vi "Collection demo.vi"() -> ()   [LabVIEW 2009]
uses:
  Minus/Minus.lvclass
  Collection.lvclass
  DAQ/DAQmx Analog.lvclass
  Lockin/Lockin SR830.lvclass
  Std Dev/Std Dev.lvclass
panel:
  out "error out":errorcluster
  in  "stop":bool
  out "Waveform Chart":waveform(dbl)[](graph)
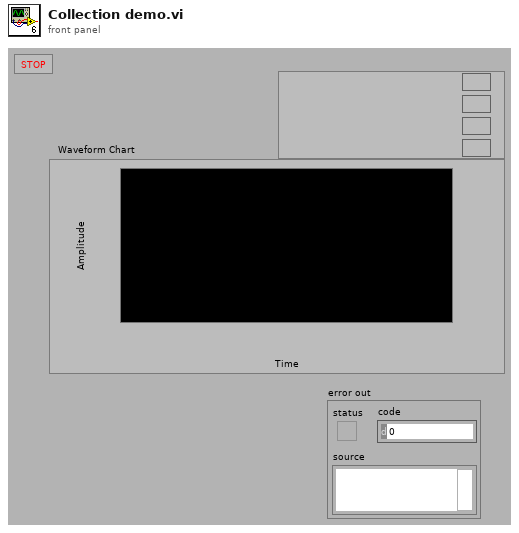
[diagram p1: front panel]
types:
  T1 = typedef "Readable.lvclass/TX Graph.ctl" = cluster{"Data Points":cluster{"t":timestamp, "x":dbl}[]}[]
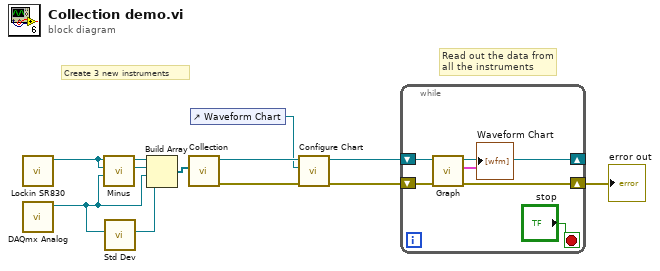
[diagram p0: block diagram]
diagram:
  # "Read out the data from\nall the instruments"
  # "Create 3 new instruments"
  n1 = call "Lockin SR830.vi"() -> ("Lockin SR830 out"=w3:refnum<class "Lockin SR830.lvclass">)  [unwired: 1 in, 10 out]
  n2 = call "DAQmx Analog.vi"() -> ("DAQmx Analog out"=w2:refnum<class "DAQmx Analog.lvclass">)  [unwired: 1 in, 10 out]
  n3 = call "Minus.vi"("Readable B"=w2, "Readable A"=w3) -> ("Minus.lvclass out"=w4:refnum<class "Minus.lvclass">)  [unwired: 1 in, 8 out]
  n4 = call "Std Dev.vi"("From"=w2) -> ("Std Dev.lvclass out"=w1:refnum<class "Std Dev.lvclass">)  [unwired: 1 in, 9 out]
  n5 = Build Array(w3, w4, w2, w1) -> (w11:refnum<class "Readable.lvclass">[])
  n6 = call "Collection.vi"("Array"=w11) -> ("error out"=w8:errorcluster, "Collection.lvclass out"=w10:refnum<class "Collection.lvclass">)  [unwired: 2 in, 7 out]
  n7 = control-ref of="Waveform Chart"() -> (w9:refnum<vi>)
  n8 = call-dynamic "Configure Chart.vi"("error in (no error)"=w8, "Waveform Chart"=w9, "Collection in"=w10) -> ("error out"=w6:errorcluster, "Collection out"=w7:refnum<class "Collection.lvclass">)  [unwired: 7 out]
  n9 = while {
    shift-right: [w16] -> _
    shift-left: w7 -> [w15]
    shift-right: [w13] -> w5
    shift-left: w6 -> [w14]
    stop <- "stop" stop-if-true
    n10 = call-dynamic "Graph.vi"("error in (no error)"=w14, "Collection in"=w15) -> ("error out"=w13:errorcluster, "History Buffers"=→"Waveform Chart":T1, "Collection out"=w16:refnum<class "Collection.lvclass">)  [unwired: 3 in, 4 out]
  }
  "error out" <- w5
